vi "turn_off_global_variable.vi"() -> ()   [LabVIEW 2013]
panel:
  in  "Stop the safe way":bool
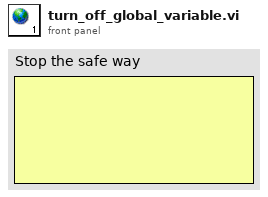
[diagram p1: front panel]
diagram:
